vi "Find RMS Velocity in_s .vi"(8 "error in (no error)":errorcluster, 11 "Y":dbl[](array[numeric])) -> (0 "error out":errorcluster, 3 "rms value":dbl)   [LabVIEW 2026, in "Acquisition.lvlib"]
uses:
  Acquisition.lvlib
  <vilib>/Analysis/3filter.llb/Filter Passband Type.ctl
  <vilib>/Analysis/5stat.llb/RMS (DBL).vi
  <vilib>/Analysis/3filter.llb/Butterworth Filter (DBL).vi
  <vilib>/Analysis/NI_AALBase.lvlib
  <vilib>/Analysis/NI_AALPro.lvlib
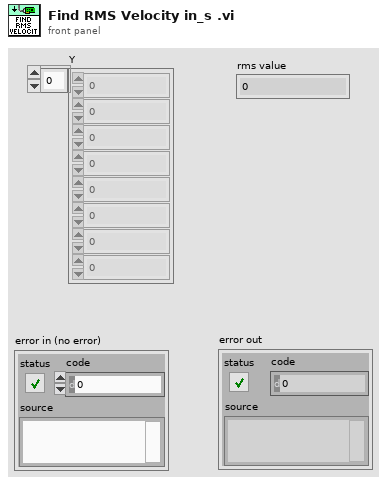
[diagram p1: front panel]
types:
  T1 = typedef "NI_AALBase.lvlib/Filter Passband Type.ctl" = enum32{"Lowpass", "Highpass", "Bandpass", "Bandstop"}
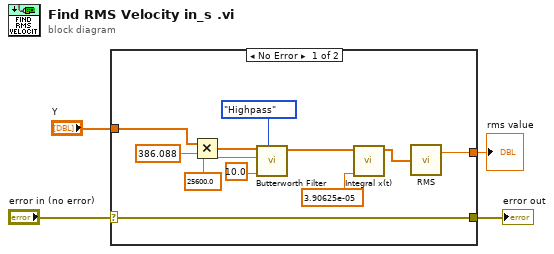
[diagram p0: block diagram]
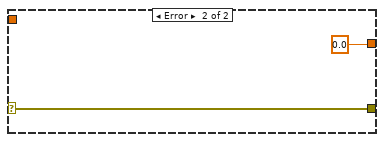
[diagram p2: hidden frame]
diagram:
  n1 = case shown="No Error" "error in (no error)" {
    selector: "error in (no error)" -> [w8 w17]
    tunnel: "Y" -> [w14 _]
    tunnel: [w8 w17] -> w2
    tunnel: [w6 0.0] -> w1
    frame No Error {
      n2 = Multiply(x=w14, y=386.088) -> (x*y=w10:dbl[])
      n3 = call-poly <vilib>:"Butterworth Filter.vi"("filter type"=Filter_Passband_Type."Highpass", "low cutoff freq: fl"=10.0 ("high cutoff freq: fh"), "sampling freq: fs"=25600.0, "X"=w10) -> ("Filtered X"=w9:dbl[])  [unwired: 4 in, 1 out]
      n4 = call <vilib>:"Integral x(t).vi"("dt"=3.90625e-05, "X"=w9) -> ("Integral X"=w7:dbl[])  [unwired: 8 in, 1 out]
      n5 = call-poly <vilib>:"RMS.vi"("X"=w7) -> ("rms value"=w6:dbl)  [unwired: 1 out]
    }
    frame Error {
    }
  }
  "error out" <- w2
  "rms value" <- w1
